vi "Color to Luminance.vi"(1 "Background Color":u32(colorbox)) -> (0 "Luminance":dbl)   [LabVIEW 2021]
doc: "Convert the color box input into the luminance calculation.\n\n<b>Code Developed By:</b>\nTechnology Service Corporation\n1983 S Liberty Drive\nBloomington, IN 47403\nPhone: 812 558-7100\ncustomtest.tsc.com\n\nDeveloper:\nDaniel Coons"
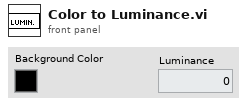
[diagram p1: front panel]
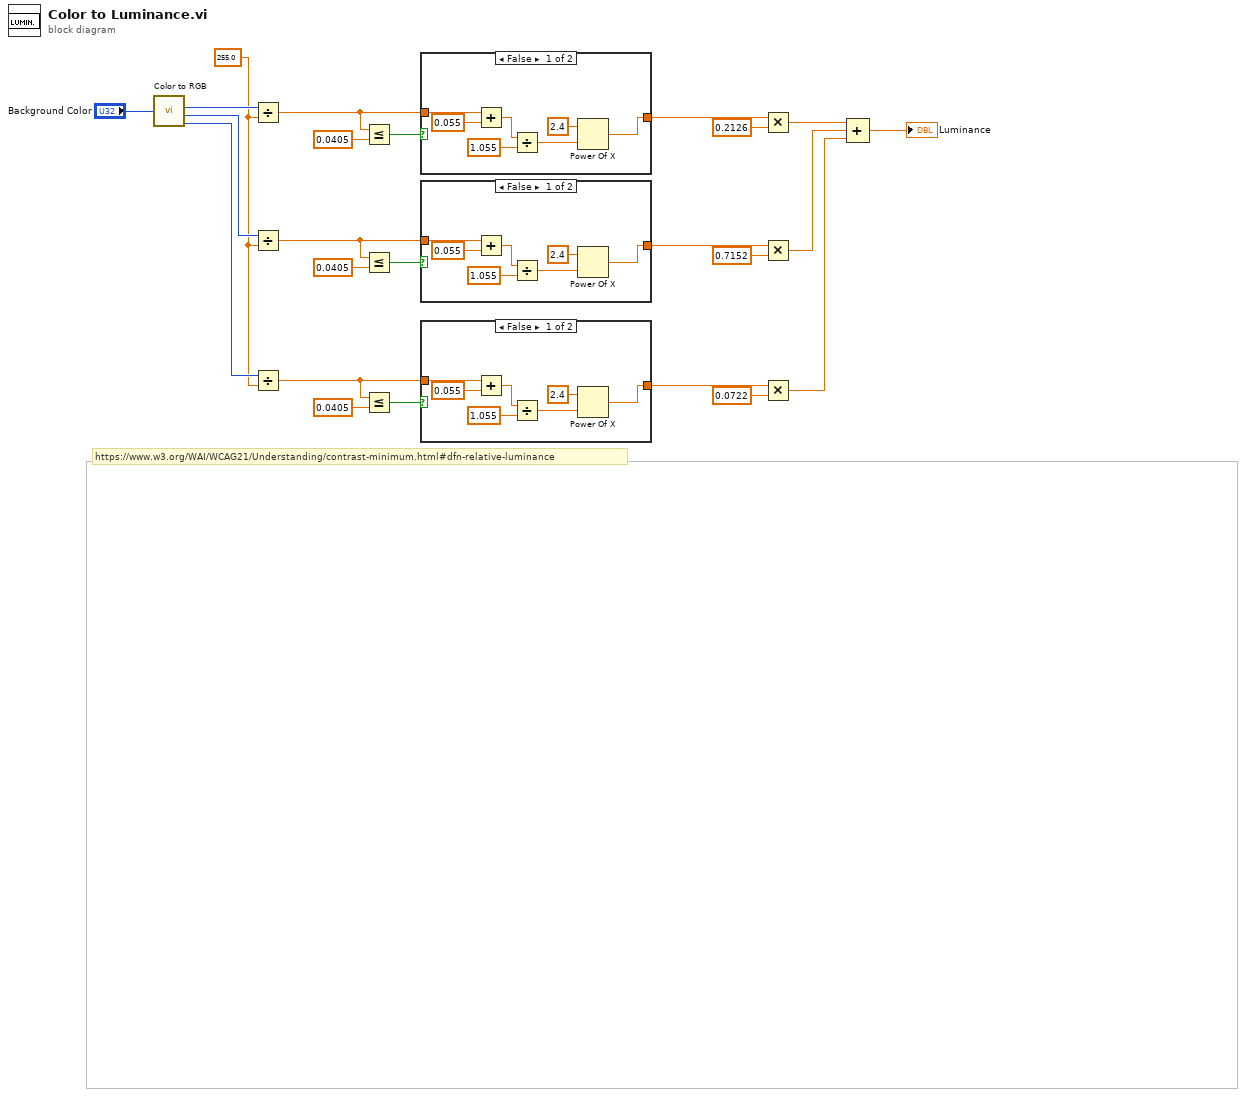
[diagram p0: block diagram]
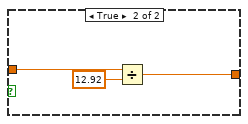
[diagram p2: hidden frame]
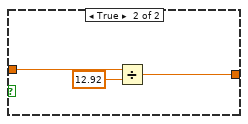
[diagram p3: hidden frame]
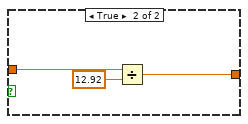
[diagram p4: hidden frame]
diagram:
  w2 = 255.0 ("y")
  # "https://www.w3.org/WAI/WCAG21/Understanding/contrast-minimum.html#dfn-relative-luminance"
  n1 = call <vilib>:"Color to RGB.vi"("Color"="Background Color") -> ("R"=w3:u8, "G"=w4:u8, "B"=w5:u8)  [unwired: 1 out]
  n2 = Divide(x=w3, y=w2) -> (x/y=w8:dbl)
  n3 = Divide(x=w4, y=w2) -> (x/y=w18:dbl)
  n4 = Divide(x=w5, y=w2) -> (x/y=w21:dbl)
  n5 = Less Or Equal?(x=w8, y=0.0405) -> (x <= y?=w7:bool)
  n6 = Less Or Equal?(x=w18, y=0.0405) -> (x <= y?=w19:bool)
  n7 = Less Or Equal?(x=w21, y=0.0405) -> (x <= y?=w22:bool)
  n8 = case shown="False" w7 {
    tunnel: w8 -> [w31 w34]
    tunnel: [w26 w32] -> w11
    frame False {
      n9 = Add(x=w31, y=0.055) -> (x+y=w29:dbl)
      n10 = Divide(x=w29, y=1.055) -> (x/y=w27:dbl)
      n11 = Power Of X(1:w27, 2:2.4 ("x")) -> (0:w26:dbl)
    }
    frame True {
      n12 = Divide(x=w34, y=12.92) -> (x/y=w32:dbl)
    }
  }
  n13 = case shown="False" w19 {
    tunnel: w18 -> [w41 w44]
    tunnel: [w36 w42] -> w20
    frame False {
      n14 = Add(x=w41, y=0.055) -> (x+y=w39:dbl)
      n15 = Divide(x=w39, y=1.055) -> (x/y=w37:dbl)
      n16 = Power Of X(1:w37, 2:2.4 ("x")) -> (0:w36:dbl)
    }
    frame True {
      n17 = Divide(x=w44, y=12.92) -> (x/y=w42:dbl)
    }
  }
  n18 = case shown="False" w22 {
    tunnel: w21 -> [w51 w54]
    tunnel: [w46 w52] -> w23
    frame False {
      n19 = Add(x=w51, y=0.055) -> (x+y=w49:dbl)
      n20 = Divide(x=w49, y=1.055) -> (x/y=w47:dbl)
      n21 = Power Of X(1:w47, 2:2.4 ("x")) -> (0:w46:dbl)
    }
    frame True {
      n22 = Divide(x=w54, y=12.92) -> (x/y=w52:dbl)
    }
  }
  n23 = Multiply(x=w11, y=0.2126) -> (x*y=w15:dbl)
  n24 = Multiply(x=w20, y=0.7152) -> (x*y=w16:dbl)
  n25 = Multiply(x=w23, y=0.0722) -> (x*y=w17:dbl)
  n26 = Compound Arithmetic op=ADD(w15, w16, w17) -> (→"Luminance":dbl)
